vi "Golander pump(mL per s, mL per rev).vi"(4 "State":i16, 5 "Time":dbl format="%.2f", 6 "Sensor Values":dbl[](array[numeric]), 7 "Set Points":dbl[](array[numeric])=[12.0, 1.0, 1.0, 1.0]) -> (0 "required data":T4={"Set Point names"=["com port", "pump address", "on state (-1=all, 167= states 1, 6, 7)", "pump (mL/rev)", "flow (mL/s)"], "required number of setpoints"=5, "required number of sensors"=0, "Sensor names"=[]}, 3 "output value":dbl)   [LabVIEW 2019]
uses:
  ProgramData/ProCoDA/Functions/Modbus devices/Pump.ctl
  Pump updates.ctl
  modbusrtu/MB Serial Master Query Write Multiple Registers (poly).vi
panel:
  out "Pump updates":T1[](array[typedef]) {"Update Time" format="%.2f"}
  in  "Pump updates":T1 {"Update Time" format="%.2f"}
  in  "Timeout":u32=120
  in  "write interval (s)":dbl=5.0
  out "pump cmd array":T2[](array[typedef])
  out "output cluster":T3
  in  "Pump cmds":T2
  in  "error in (no error)":errorcluster
  out "VISA out":refnum<visa-resource-name>
  out "error out":errorcluster
  # "failure at 80 ms"
  # "Enter the correct information for this control code in the required data structure below. Then make the current value default by right clicking on the border of the data structure. Select \"data operations\" and then select \"make current value default\". These values will be displayed by process controller."
  # "Mode: RTU\nAddresses: 1-247 (User Defined)\nBaud Rate: 9600\nData Bits: 8\nCRC: Even Parity\nStop Bit: 1"
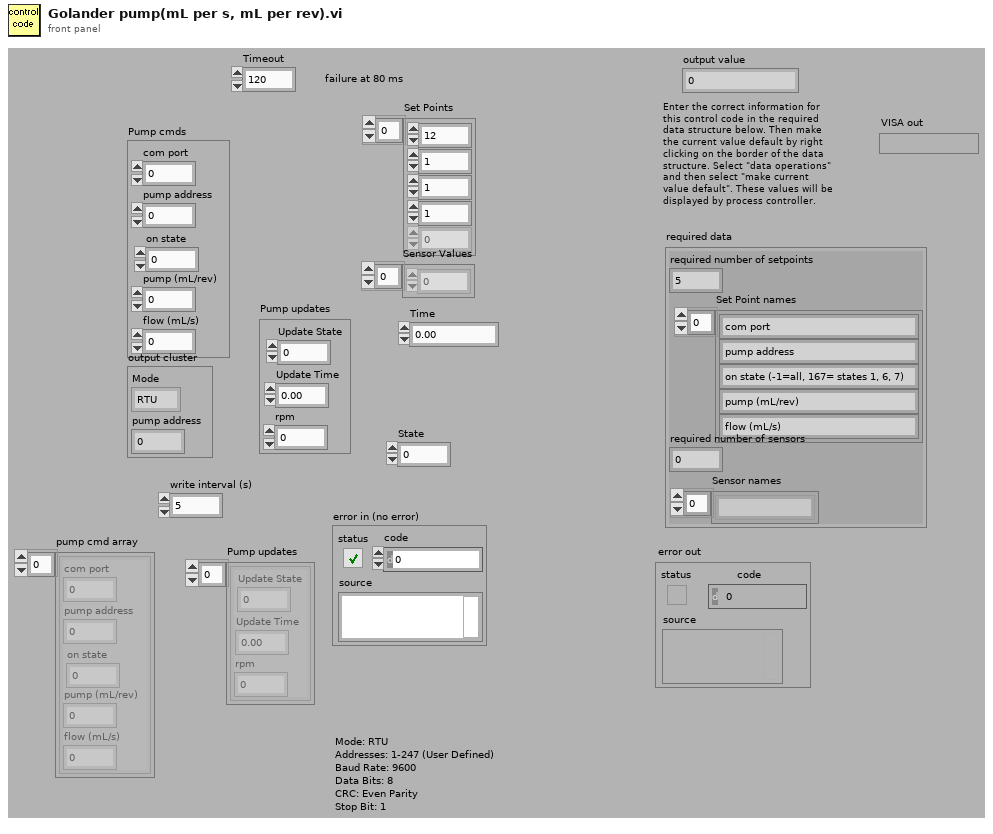
[diagram p1: front panel]
types:
  T1 = typedef "Pump updates.ctl" = cluster{"Update State":i16, "Update Time":dbl, "rpm":dbl}
  T2 = typedef "Pump.ctl" = cluster{"com port":u8, "pump address":u8, "on state":i32, "pump (mL/rev)":dbl, "flow (mL/s)":dbl}
  T3 = cluster{"Mode":enum16{"RTU", "ASCII"}, "pump address":u8}
  T4 = cluster{"Set Point names":string[], "required number of setpoints":u8, "required number of sensors":u8, "Sensor names":string[]}
  T5 = cluster{"Set Points[0]":dbl, "Set Points[1]":dbl, "Set Points[2]":dbl, "Set Points[3]":dbl, "Set Points[4]":dbl}
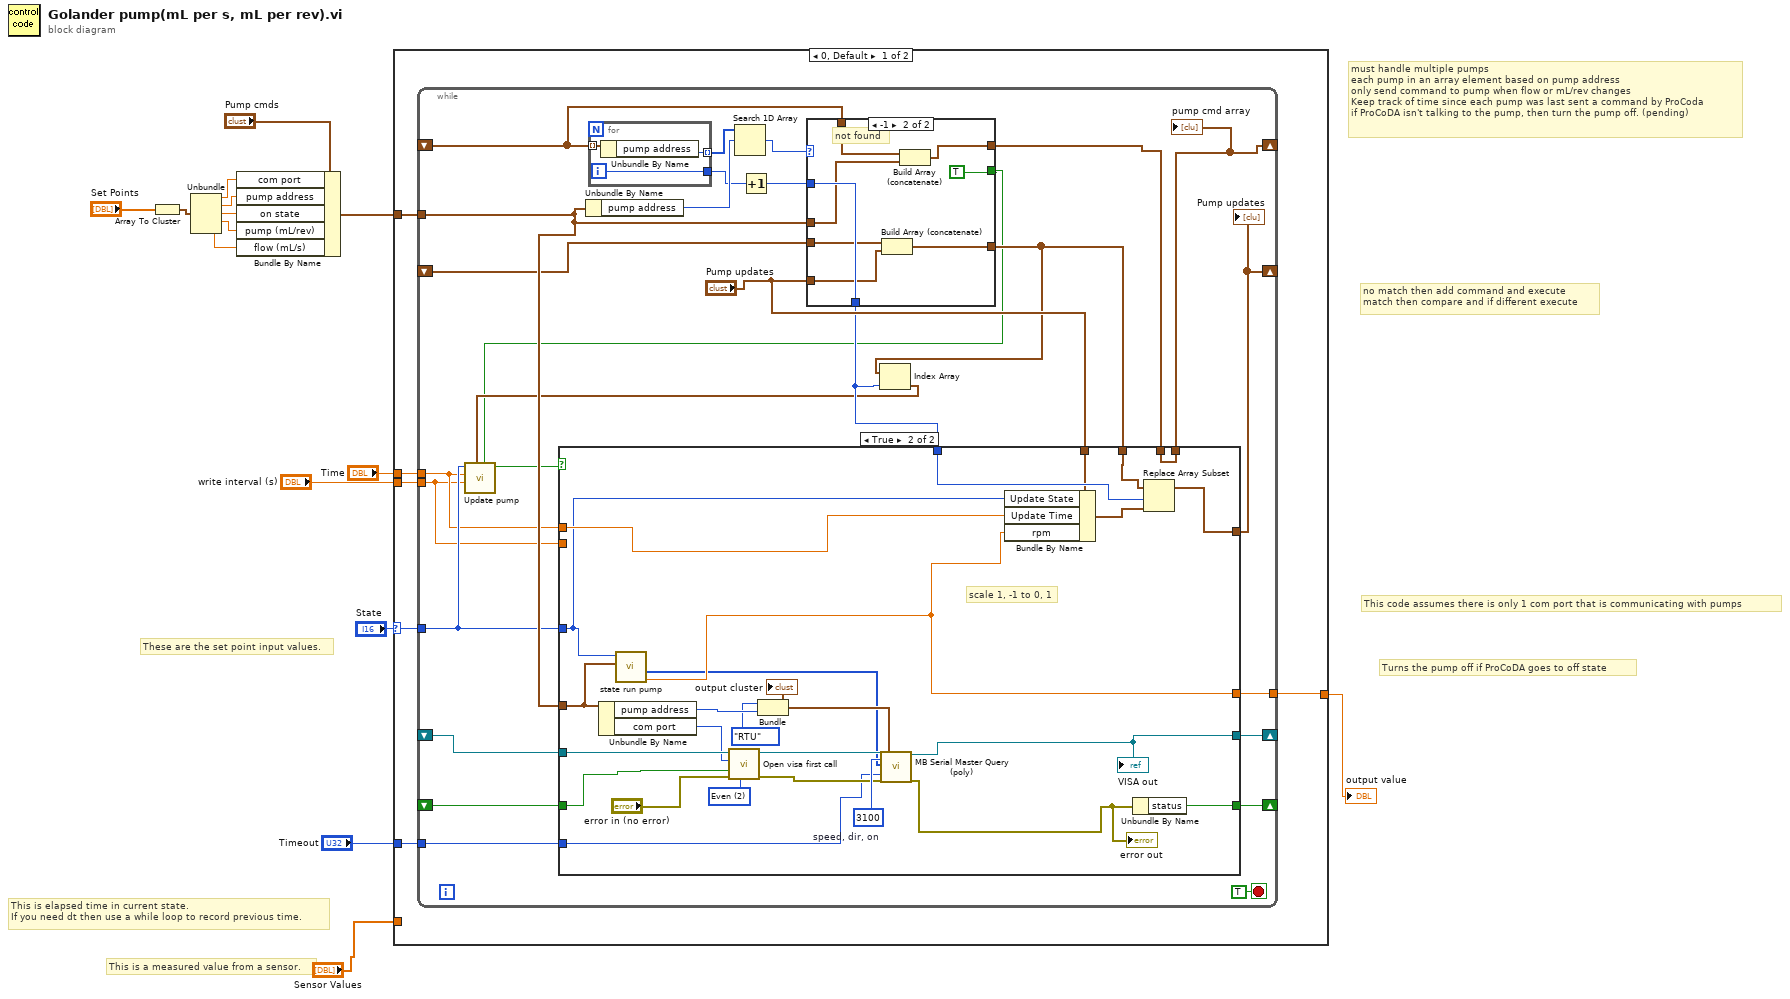
[diagram p0: block diagram]
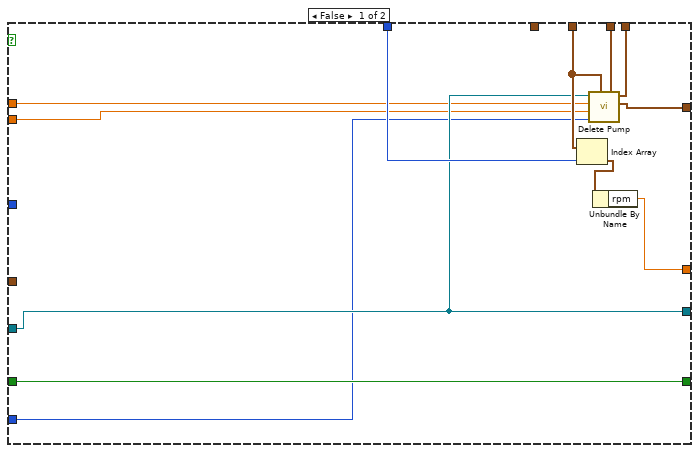
[diagram p2: hidden frame]
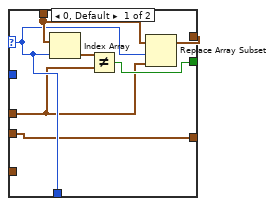
[diagram p3: hidden frame]
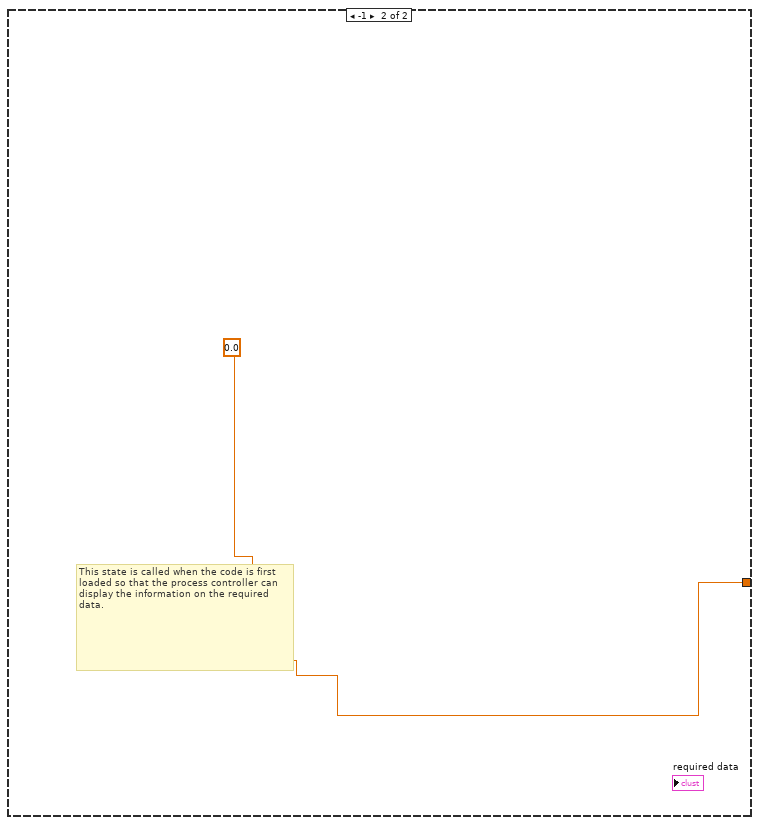
[diagram p4: hidden frame]
diagram:
  # "Turns the pump off if ProCoDA goes to off state"
  # "This code assumes there is only 1 com port that is communicating with pumps"
  # "no match then add command and execute\nmatch then compare and if different execute"
  # "must handle multiple pumps\neach pump in an array element based on pump address\nonly send command to pump when flow or mL/rev changes\nKeep track of time since each pump was last sent a command by ProCoda\nif ProCoDA isn't talking to the pump, then turn the pump off. (pending)"
  # "These are the set point input values."
  # "This is a measured value from a sensor."
  # "This is elapsed time in current state.\nIf you need dt then use a while loop to record previous time."
  n1 = Array To Cluster(array="Set Points") -> (cluster=w12:T5)
  n2 = Unbundle(w12) -> ("Set Points[0]"=w8:dbl, "Set Points[1]"=w13:dbl, "Set Points[2]"=w3:dbl, "Set Points[3]"=w5:dbl, "Set Points[4]"=w4:dbl)
  n3 = Bundle By Name(cluster="Pump cmds", "com port"=w8, "pump address"=w13, "on state"=w3, "pump (mL/rev)"=w5, "flow (mL/s)"=w4) -> (w10:T2)
  n4 = case shown="0, Default" "State" {
    selector: "State" -> [w19 _]
    tunnel: [w20 0.0 ("fraction on")] -> w7
    tunnel: w10 -> [w21 _]
    tunnel: "Sensor Values" -> [_ _]
    tunnel: "Time" -> [w18 _]
    tunnel: "write interval (s)" -> [w17 _]
    tunnel: "Timeout" -> [w16 _]
    frame 0, Default {
      n5 = while {
        shift-right: [w44] -> _
        shift-left: _ -> [w47]
        tunnel: w21 -> [w36]
        shift-right: [w45] -> _
        shift-left: _ -> [w46]
        shift-right: [w23] -> _
        shift-left: _ -> [w39]
        tunnel: w19 -> [w30]
        tunnel: w18 -> [w29]
        shift-right: [w34] -> _
        shift-left: _ -> [w35]
        tunnel: w17 -> [w22]
        tunnel: [w43] -> w20
        tunnel: w16 -> [w25]
        stop <- TRUE stop-if-true
        n6 = Unbundle By Name(w36) -> ("pump address"=w41:u8)
        n7 = for {
          tunnel: [w104] -> w42 mode=indexing
          tunnel: w39 -> [w103] mode=indexing
          tunnel: [w102] -> w38
          i -> [w102]
          n8 = Unbundle By Name(w103) -> ("pump address"=w104:u8)
        }
        n9 = Search 1D Array(1D array=w42, element=w41) -> (index of element=w40:i32)  [unwired: 1 in]
        n10 = Increment(x=w38) -> (x+1=w37:i32)
        n11 = case shown="-1" w40 {
          selector: w40 -> [w89 _]
          tunnel: [w92 TRUE] -> w26
          tunnel: w39 -> [w91 w100]
          tunnel: [w90 w99] -> w24
          tunnel: w37 -> [_ w98]
          tunnel: [w89 w98] -> w32
          tunnel: w36 -> [w88 w97]
          tunnel: w35 -> [w87 w96]
          tunnel: [w87 w95] -> w31
          tunnel: "Pump updates" -> [_ w94]
          frame 0, Default {
            n12 = Index Array(array=w91, index=w89) -> (element=w93:T2)
            n13 = Not Equal?(x=w93, y=w88) -> (x != y?=w92:bool)
            n14 = Replace Array Subset(array=w91, new element=w88, index=w89) -> (w90:T2[])
          }
          frame -1 {
            # "not found"
            n15 = Build Array (concatenate)(w96, w94) -> (w95:T1[])
            n16 = Build Array (concatenate)(w100, w97) -> (w99:T2[])
          }
        }
        n17 = Index Array(array=w31, index=w32) -> (element=w28:T1)
        n18 = call "Update pump.vi"("new pump cmd"=w26, "Pump updates"=w28, "write interval (s)"=w22, "Time"=w29, "State"=w30) -> ("update"=w27:bool)  [unwired: 6 in]
        n19 = case shown="True" w27 {
          tunnel: w47 -> [w52 w85]
          tunnel: w46 -> [w60 w61]
          tunnel: [w60 w84] -> w45
          tunnel: [w52 w64] -> w44
          tunnel: [w57 w66] -> w43
          tunnel: w36 -> [_ w73]
          tunnel: w30 -> [_ w65]
          tunnel: w29 -> [w51 w70]
          tunnel: [w55 w74] -> w34
          tunnel: w31 -> [w56 w75]
          tunnel: w32 -> [w59 w71]
          tunnel: "Pump updates" -> [_ w69]
          tunnel: w25 -> [w50 w68]
          tunnel: w24 -> [w54 w67]
          tunnel: [w53 w67] -> w23
          tunnel: w22 -> [w49 _]
          frame False {
            n20 = Index Array(array=w56, index=w59) -> (element=w58:T1)
            n21 = call "Delete Pump.vi"("pump cmd array"=w54, "Pump updates"=w56, "Timeout"=w50, "write interval (s)"=w49, "Time"=w51, "VISA"=w52) -> ("Pump updates out"=w55:T1[], "pump cmd array out"=w53:T2[])  [unwired: 4 in]
            n22 = Unbundle By Name(w58) -> ("rpm"=w57:dbl)
          }
          frame True {
            w76 = u16 2 items=["None", "Odd", "Even", "Mark", "Space"] ("Parity")
            w79 = u16 3100  # speed, dir, on
            # "scale 1, -1 to 0, 1"
            n23 = Unbundle By Name(w73) -> ("pump address"=w81:u8, "com port"=w83:u8)
            n24 = call "state run pump.vi"("pump command"=w73, "State"=w65) -> ("rpm"=w66:dbl, "registers"=w62:u16[])  [unwired: 2 in, 2 out]
            n25 = call "Open visa first call.vi"("Parity"=w76, "error in (no error)"="error in (no error)", "error"=w61, "Com port"=w83, "VISA Refnum in"=w85) -> ("error out"=w78:errorcluster, "VISA Refnum out"=w82:refnum<visa-resource-name>)  [unwired: 5 in]
            n26 = Bundle("Mode"=enum16{"RTU", "ASCII"}."RTU", "pump address"=w81) -> (w77:T3)  [unwired: 1 in]
            "output cluster" <- w77
            n27 = call-poly "MB Serial Master Query (poly).vi"("VISA resource name"=w82, "Starting Address"=w79, "Registers"=w62, "Timeout"=w68, "error in"=w78, "Serial Parameters"=w77) -> ("VISA resource name out"=w64:refnum<visa-resource-name>, "error out"=w63:errorcluster)  [unwired: 11 in, 1 out]
            "VISA out" <- w64
            "error out" <- w63
            n28 = Bundle By Name(cluster=w69, "Update State"=w65, "Update Time"=w70, "rpm"=w66) -> (w72:T1)
            n29 = Unbundle By Name(w63) -> ("status"=w84:bool)
            n30 = Replace Array Subset(array=w75, new element=w72, index=w71) -> (w74:T1[])
          }
        }
        "pump cmd array" <- w23
        "Pump updates" <- w34
      }
    }
    frame -1 {
      # "This state is called when the code is first loaded so that the process controller can display the information on the required data."
    }
  }
  "output value" <- w7
